vi "CsTool-ConfigureAcquisitionAll.vi"(0 "Handle Cluster":T2, 1 "Segment Count (1)":u32=1, 2 "Acquisition":T1={"Sample Rate"=100000000.0, "Clock Mode"=enum."Internal", "Mode"="Dual", "Depth"=8192.0, "Segment Size"=8192.0, "Trigger Timeout"=1000000.0, "Trigger Holdoff"=0.0, "Trigger Delay"=0.0}, 3 "Invert Clock (f)":bool, 4 "Extended Options (0)":i32) -> (5 "Error Code":i32)   [LabVIEW 2022 SP3]
doc: "This VI sends the requested Acquisition configuration settings to the driver for the system identified by Handle Cluster, which is obtained by using CsTool-GetSystem.vi. The requested settings are not actually sent to the CompuScope hardware until CsTool-Commit.vi is called. \n\nThe Acquisition cluster settings are Sample Rate, Clock Mode, Mode, Depth, Segment Size, Trigger Timeout, Trigger Delay, and Trigger Holdoff. There are also the Segment Count, Invert Clock and Extended Options input settings. Valid values for the system identified by Handle Cluster must be supplied for all settings. If no connection is made to an input, the default value for that input will be used. \n\nIf the VI fails, an appropriate error code is returned in the Error Code indicator. A descriptive error string may be obtained by calling CsTool-ErrorHandler.vi.\n\n\nInput Value Descriptions:\n\nSample Rate (default = 100000000)\nThis double variable value is the rate, in samples per second, at which the CompuScope system will sample input signals. If the desired sampling rate is not valid for the CompuScope system identified by the Handle Cluster, an appropriate error code is returned.\n\nClock Mode (default = Internal)\nThis Enum value defines the clock mode of the CompuScope system. Valid values are Internal, External or Reference. If an external clock is being used, the rate entered in the Sample Rate field must be set to the correct external clock signal frequency. Reference clock mode means that the internal oscillator will be synchronized with a 10 MHz reference clock that is connected to the external clock input. If Internal is selected, the Sample Rate field selects the frequency of the internal oscillator. Note: The Reference clock mode is not supported by all CompuScope models.\n\nMode (default = Dual)\nThis string sets the operating mode for the CompuScope system. Available modes for most CompuScope cards are Single and Dual. Some newer models also have Quad and Octal modes. Digital input CompuScope cards, like the CS3200, may be set to 8-bit, 16-bit, or 32-bit modes. If the requested mode is invalid for the CompuScope system, an appropriate error code is returned.\n\nDepth (default =8192)\nThis double variable value is the number of post-trigger samples that the CompuScope system will acquire after the occurrence of the trigger event. \n\nSegment Size (default = 8192)\nThis double variable controls the total amount of memory allocated to the acquisition. The maximum possible amount of pre-trigger data that can be acquired, therefore, is (Segment Size - Depth). \n\nTrigger Timeout (default = 1000000)\nThis double variable value is the amount of time, in microseconds, that the CompuScope system will wait for a trigger to occur before forcing a trigger. An input value of -1 indicates no trigger timeout, so that the CompuScope system will wait forever for a trigger event.\n\nTrigger Delay (default = 0)\nThis double variable value is the duration, in Samples, between the time that the trigger event actually occurs and the time that the trigger event will be logged in the data record. Setting a non-zero trigger delay is useful for signals where the region of interest in the signal occurs long after the trigger event. Trigger Delay is not supported on all CompuScope models. If the CompuScope system identified by Handle Cluster does not support Trigger Delay, this value will be ignored.\n\nTrigger Holdoff (default = 0)\nThis double variable value is the number of samples during which the CompuScope hardware will ignore trigger events after starting an acquisition. Trigger Holdoff is useful in order to ensure the accumulation of a specified number of pre-trigger points. This is achieved by ignoring trigger events until the specified number of pre-trigger points has been acquired.\n\nSegment Count (default = 1)\nThis integer value sets how many segments (or records) will be acquired in a Multiple Record acquisition. For Single Record acquisitions, Segment Count must be set to 1.\n\nInvert Clock (default = FALSE)\nWhen TRUE, this Boolean value inverts the external clock supplied to a digital input CompuScope cards, like the CS3200, so that it samples on the falling edge of the clocking signal rather than on the rising edge. This setting is ignored on analog input CompuScope cards."
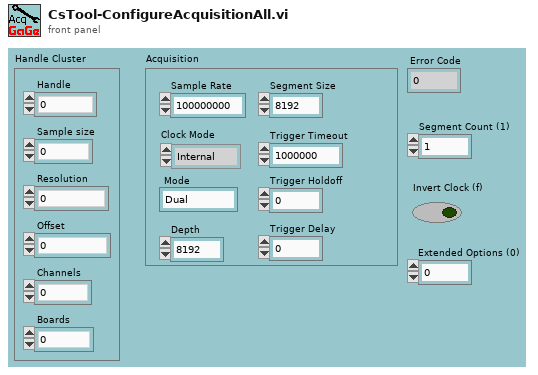
[diagram p1: front panel]
types:
  T1 = cluster{"Sample Rate":dbl, "Clock Mode":enum16{"Internal", "External", "Reference"}, "Mode":string, "Depth":dbl, "Segment Size":dbl, "Trigger Timeout":dbl, "Trigger Holdoff":dbl, "Trigger Delay":dbl}
  T2 = cluster{"Handle":u32, "Sample size":u32, "Resolution":i32, "Offset":i32, "Channels":u32, "Boards":u32}
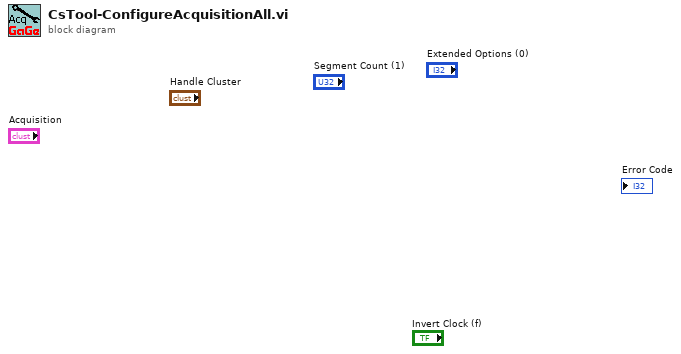
[diagram p0: block diagram]
diagram:
